vi "SYST_UPR.vi"(0 "VISA IN":refnum<visa-resource-name>, 5 "error in":errorcluster) -> (14 "VISA Out":refnum<visa-resource-name>, 19 "error out":errorcluster)   [LabVIEW 2018, in "PNA-X.lvlib"]
doc: "SYSTem:UPReset \n(Write-only) Performs a User Preset. There must be an active User Preset state file (see Load and \nSave) or an error will be returned. Learn more about User Preset. \nRegardless of the state of the User Preset Enable checkbox, the SYST:PRESet command will always \npreset the PNA to the factory preset settings, and SYST:UPReset will always perform a User Preset. \nExamples SYST:UPReset \nsystem:upreset \nQuery Syntax Not Applicable \nDefault Not Applicable"
uses:
  PNA-X.lvlib
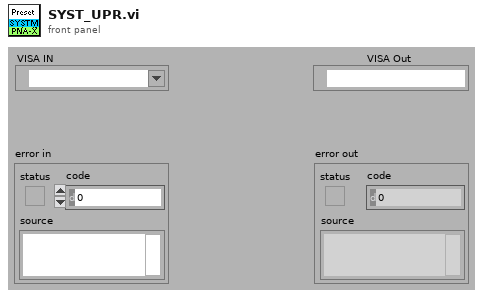
[diagram p1: front panel]
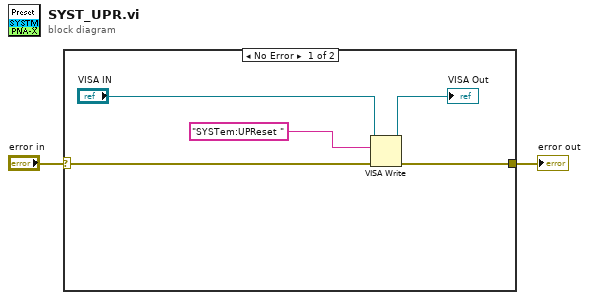
[diagram p0: block diagram]
diagram:
  n1 = case shown="No Error" "error in" {
    selector: "error in" -> [w3 w8]
    tunnel: [w6 w8] -> w1
    frame No Error {
      n2 = VISA Write(VISA resource name="VISA IN", write buffer="SYSTem:UPReset " ("Cmdline"), error in (no error)=w3) -> (VISA resource name out=→"VISA Out":refnum<visa-resource-name>, error out=w6:errorcluster)  [unwired: 1 out]
    }
    frame Error {
    }
  }
  "error out" <- w1
